vi "Protocol Write.vi"(8 "error in (no error)":errorcluster, 9 "timeout":i32=10000, 10 "data":u8[](array[numeric]), 11 "protocol layer in":refnum<class "TCP Slave.lvclass">) -> (0 "error out":errorcluster, 1 "timed out?":bool, 3 "protocol layer out":refnum<class "TCP Slave.lvclass">)   [LabVIEW 2015, in "SubVIs.lvlib" / "TCP Slave.lvclass"]
doc: "Writes to the established TCP connection stored in the class."
uses:
  <vilib>/Modbus/subvis/Protocol/TCP/TCP Slave/TCP Slave.lvclass
  <vilib>/Modbus/subvis/Protocol/TCP/TCP Slave/TCP Slave.lvclass/TCP Slave.ctl
  <vilib>/Modbus/subvis/Protocol/TCP/TCP Shared Components/TCP Shared Components.lvlib
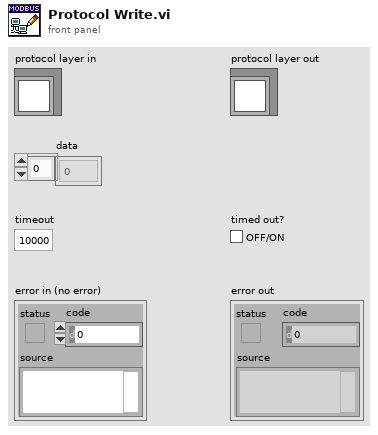
[diagram p1: front panel]
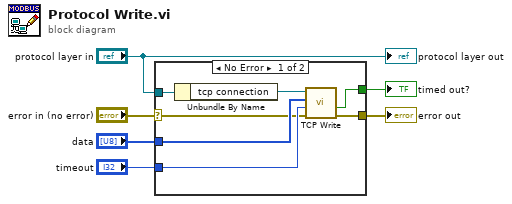
[diagram p0: block diagram]
diagram:
  n1 = case shown="No Error" "error in (no error)" {
    selector: "error in (no error)" -> [w7 w14]
    tunnel: "protocol layer in" -> [w13 _]
    tunnel: "data" -> [w11 _]
    tunnel: "timeout" -> [w10 _]
    tunnel: [w9 w14] -> w3
    tunnel: [w8 _] -> w2
    frame No Error {
      n2 = Unbundle By Name(w13) -> ("tcp connection"=w12:refnum<k5>)
      n3 = call <vilib>:"TCP Write.vi"("error in (no error)"=w7, "timeout"=w10, "data"=w11, "connection ID"=w12) -> ("error out"=w9:errorcluster, "timed out?"=w8:bool)  [unwired: 6 in]
    }
    frame Error {
    }
  }
  "error out" <- w3
  "timed out?" <- w2
  "protocol layer out" <- "protocol layer in"
